vi "Read Tree Ctl.vi"(8 "error in (no error)":errorcluster, 11 "Tree Manager in":refnum<class "Tree Manager.lvclass">) -> (0 "error out":errorcluster, 2 "Tree Ctl":refnum<vi>, 3 "Tree Manager out":refnum<class "Tree Manager.lvclass">)   [LabVIEW 2026, in "VILab.lvlib" / "Tree Manager.lvclass"]
uses:
  Tree Manager.lvclass
  Tree Manager.lvclass/Tree Manager.ctl
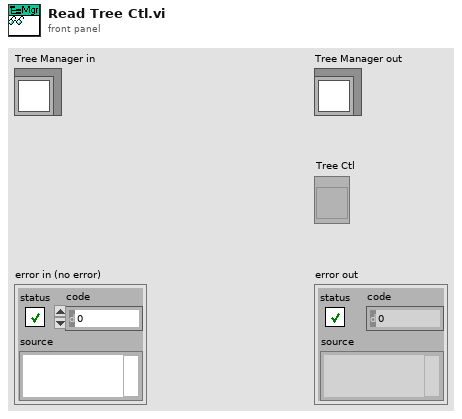
[diagram p1: front panel]
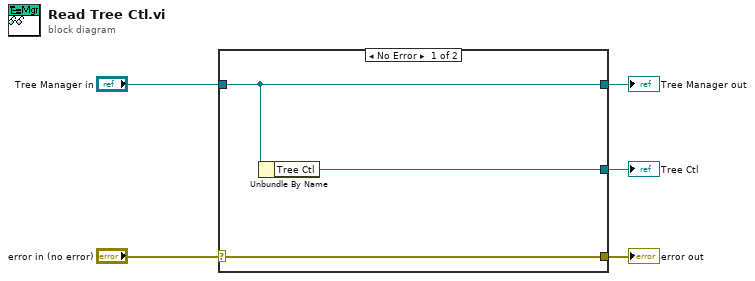
[diagram p0: block diagram]
diagram:
  n1 = case shown="No Error" "error in (no error)" {
    selector: "error in (no error)" -> [w8 w9]
    tunnel: [w8 w9] -> w4
    tunnel: [w7 w10] -> w2
    tunnel: "Tree Manager in" -> [w7 w10]
    tunnel: [w6 _] -> w1
    frame No Error {
      n2 = Unbundle By Name(w7) -> ("Tree Ctl"=w6:refnum<vi>)
    }
    frame Error {
    }
  }
  "error out" <- w4
  "Tree Manager out" <- w2
  "Tree Ctl" <- w1
